vi "AlazarDSPGetModules.vi"(0 "Handle":u64, 1 "error in (no error)":errorcluster) -> (2 "Handle":u64, 3 "Return Code":u32, 4 "DSP Modules":u64[](array[numeric]), 5 "error out":errorcluster)   [LabVIEW 2018]
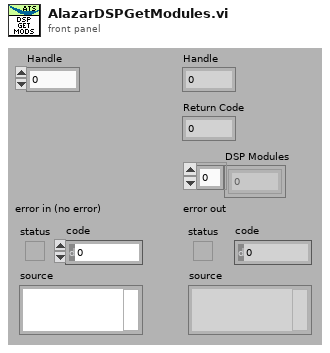
[diagram p1: front panel]
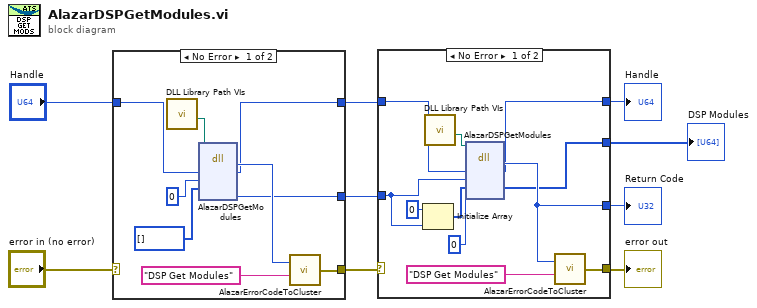
[diagram p0: block diagram]
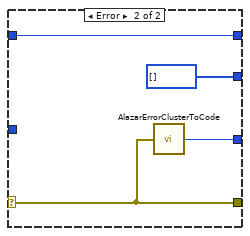
[diagram p2: hidden frame]
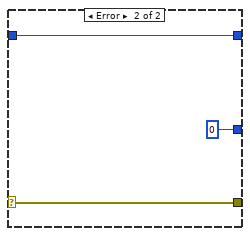
[diagram p3: hidden frame]
diagram:
  n1 = case shown="No Error" "error in (no error)" {
    selector: "error in (no error)" -> [_ w21]
    tunnel: [w15 w21] -> w1
    tunnel: "Handle" -> [w18 w20]
    tunnel: [w14 w20] -> w6
    tunnel: [w12 0] -> w7
    frame No Error {
      n2 = call "DLL Library Path VIs.vi"() -> ("Alazar"=w10:path)  [unwired: 5 in, 6 out]
      n3 = dll-call lib="C:/Project/SerialSectOCT - FFT GPU/SerialSectOCT/Labview Software/DLL/ATSApi.dll" fn="AlazarDSPGetModules"(path in=w10, "handle"=w18, "numEntries"=u32 0, "modules"=u64[] []) -> ("return type"=w17:u32, "handle"=w14:u64, "numModules"=w12:u32)  [unwired: 5 in, 2 out]
      n4 = call "AlazarErrorCodeToCluster.vi"("Message"="DSP Get Modules", "Error Code"=w17) -> ("error out"=w15:errorcluster)
    }
    frame Error {
    }
  }
  n5 = case shown="No Error" w1 {
    selector: w1 -> [_ w36]
    tunnel: [w29 w36] -> w4
    tunnel: [w31 w35] -> w5
    tunnel: w6 -> [w32 w34]
    tunnel: [w28 w34] -> w3
    tunnel: w7 -> [w27 _]
    tunnel: [w24 u32[] []] -> w2
    frame No Error {
      n6 = Initialize Array(u64 0, w27) -> (w25:u64[])
      n7 = call "DLL Library Path VIs.vi"() -> ("Alazar"=w22:path)  [unwired: 5 in, 6 out]
      n8 = dll-call lib="C:/Project/SerialSectOCT - FFT GPU/SerialSectOCT/Labview Software/DLL/ATSApi.dll" fn="AlazarDSPGetModules"(path in=w22, "handle"=w32, "numEntries"=w27, "modules"=w25, "numModules"=u32 0) -> ("return type"=w31:u32, "handle"=w28:u64, "modules"=w24:u64[])  [unwired: 4 in, 2 out]
      n9 = call "AlazarErrorCodeToCluster.vi"("Message"="DSP Get Modules", "Error Code"=w31) -> ("error out"=w29:errorcluster)
    }
    frame Error {
      n10 = call "AlazarErrorClusterToCode.vi"("error in (no error)"=w36) -> ("Error Code"=w35:u32)
    }
  }
  "Handle" <- w3
  "error out" <- w4
  "Return Code" <- w5
  "DSP Modules" <- w2
